vi "SVPWM_timing_gen.vi"(0 "ref_beta":sgl caption="voltage beta", 5 "Period":i32=1, 7 "ref_max":sgl=0.9999695, 9 "input valid":bool=TRUE, 11 "ref_alpha":sgl caption="voltage alpha") -> (4 "Sector":u8, 6 "C_Timing":cluster{"ON":u32, "OFF":u32}, 8 "B_timing":cluster{"ON":u32, "OFF":u32}, 10 "output valid":bool, 14 "feedback signals":cluster{"ready for input":bool}, 15 "A_timing":cluster{"ON":u32, "OFF":u32})   [LabVIEW 2017]
doc: "This VI is created by the NI LabVIEW 2017 FPGA IP Builder.\n\nProject: SVPWM_dev.lvproj\nTarget: FPGA Target (sbRIO-9607)/IP Builder\nBuild Specification: SVPWM_TimingGen_SGL_gen\nDirectives Item: SVPWM_TimingGen_SGL_src\nTop-Level VI: C:\\PowerElectronicControl\\SpaceVectorPWM\\dev\\IPBuilder\\SVPWM_TimingGen_SGL_src.vi\n\nQuick Device Utilization Estimate\n--------------------------------------------\nSlice Registers: 1.5% (1639 out of 106400)\nSlice LUTs: 14.4% (7651 out of 53200)\nDSP48s: 4.1% (9 out of 220)\nBlock RAMs: 1.8% (5 out of 280)\n\nQuick Performance Estimate\n--------------------------------------------\nClock rate (MHz): 45.83\nInitiation interval (cycles): 25\nPipeline type: Not pipelined\nMinimum latency: 24\nMaximum latency: 24"
uses:
  <vilib>/rvi/IPIntegrationNode/IPINode_Typedef/niFpgaIPINodeSupportedFamilies.ctl
  <vilib>/rvi/IPIntegrationNode/IPINode_Utilities/niFpgaIPINodeSimCore.vi
  <vilib>/rvi/IPIntegrationNode/IPINode_Xnode/niFpgaIPINode.xnode
  SVPWM_timing_gen Support/IPBlockSimFiles/xsim.dir/m3C5B92D4_topH/xsimk8E869ECA943C4BA0BA3461207F03B294.dll
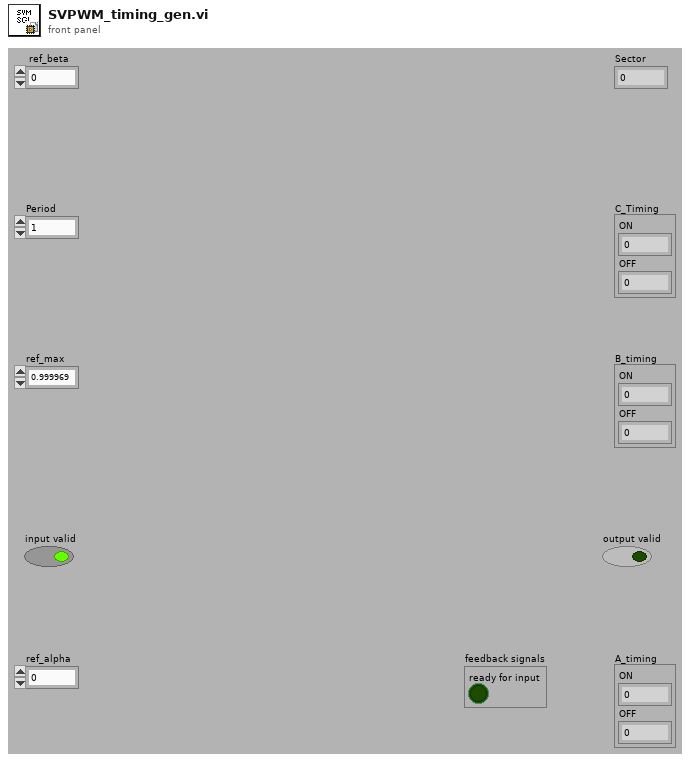
[diagram p1: front panel]
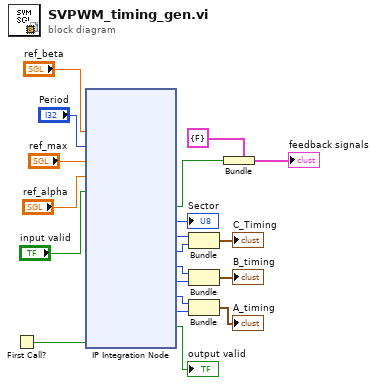
[diagram p0: block diagram]
diagram:
  n1 = First Call?() -> (First Call?: T/F=w20:bool)
  n2 = xnode "IP Integration Node"("p_5"="ref_beta", "p_2"="Period", "p_1"="ref_max", "p_0"="ref_alpha", "input_valid"="input valid", "first_call"=w20) -> ("ready_for_input"=w17:bool, "p_15"=→"Sector":u8, "p_8_e_0"=w5:u32, "p_8_e_1"=w6:u32, "p_6_e_0"=w3:u32, "p_6_e_1"=w4:u32, "p_4_e_0"=w1:u32, "p_4_e_1"=w2:u32, "output_valid"=→"output valid":bool)  [unwired: 2 in]
  n3 = Bundle("p_8_e_0"=w5, "p_8_e_1"=w6) -> (→"C_Timing":cluster{"p_8_e_0":u32, "p_8_e_1":u32})  [unwired: 1 in]
  n4 = Bundle("p_6_e_0"=w3, "p_6_e_1"=w4) -> (→"B_timing":cluster{"p_6_e_0":u32, "p_6_e_1":u32})  [unwired: 1 in]
  n5 = Bundle("p_4_e_0"=w1, "p_4_e_1"=w2) -> (→"A_timing":cluster{"p_4_e_0":u32, "p_4_e_1":u32})  [unwired: 1 in]
  n6 = Bundle ("Bundle_feedback")(cluster=cluster{"ready for input":bool} {"ready for input"=FALSE}, "ready for input"=w17) -> (→"feedback signals":cluster{"ready for input":bool})
